vi "Zuordnungstabelle Spaltenbezeichnungen.vi"(11 "Anzahl der Stellungen (10)":i16=10) -> (3 "Spaltenbezeichnungen":string[](array[string]))   [LabVIEW 2020, in "Anlagenuebersicht.lvlib" / "VisBx Anzeige.lvlib"]
doc: "Die Zuordnungstabelle hat für jede Prozessvariable eine Zeile und enthält in\n\nSpalte 0 (Stellung x):\nden bisherigen Wert der Variablen, der zB. der Stellung eines Ventils entspricht (Boolean, U8 oder Enum),\nbei Ziffernanzeigen (U16, I16, ... DBL) immer Null.\n\nSpalte 1 (steuernd):\ndie Variablen-Nummer N einer anderen Prozessvariablen, welche die Parameter einer Ziffernanzeige festlegt (steuerndes N vom Typ Boolean, U8 oder Enum). Wenn keine Steuerung der Parameter verwendet wird, ist der Wert -1.\n\nSpalte 2 (Nachkomma):\ndie Anzahl der Nachkommastellen beim Datentyp DBL, sonst 0.\n\nSpalte 3 (Stellungstyp):\n0 ... kein Stellungstyp, zB. Ziffernanzeige\n1 ... Stellungstyp (Boolean, U8 oder Enum)\n\nSpalte 4: Programmindex für x=0\nSpalte 5: Anzahl der Programm-Schritte für x=0\n\nSpalte 6: Programmindex für x=1\nSpalte 7: Anzahl der Programm-Schritte für x=1\n....\n....\nSpalte 22: Programmindex für x=9\nSpalte 23: Anzahl der Programm-Schritte für x=9"
uses:
  VisBx Anzeige.lvlib
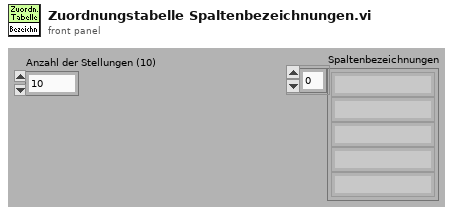
[diagram p1: front panel]
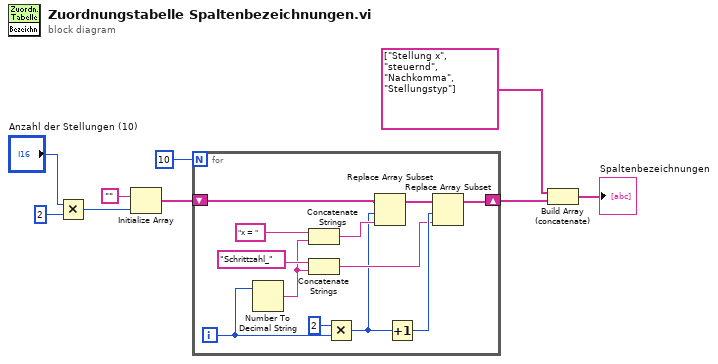
[diagram p0: block diagram]
diagram:
  n1 = Multiply(x="Anzahl der Stellungen (10)", y=i16 2) -> (x*y=w1:i16)
  n2 = Initialize Array("", w1) -> (w8:string[])
  n3 = for {
    N: 10 -> [_]
    shift-right: [w11] -> w5
    shift-left: w8 -> [w18]
    i -> [w15]
    n4 = Number To Decimal String(number=w15) -> (decimal integer string=w19:string)  [unwired: 1 out]
    n5 = Concatenate Strings("x = ", w19) -> (w13:string)
    n6 = Concatenate Strings("Schrittzahl_", w19) -> (w12:string)
    n7 = Multiply(x=2, y=w15) -> (x*y=w10:i32)
    n8 = Replace Array Subset(array=w18, new element=w13, index=w10) -> (w17:string[])
    n9 = Increment(x=w10) -> (x+1=w16:i32)
    n10 = Replace Array Subset(array=w17, new element=w12, index=w16) -> (w11:string[])
  }
  n11 = Build Array (concatenate)(string[] ["Stellung x", "steuernd", "Nachkomma", "Stellungstyp"], w5) -> (→"Spaltenbezeichnungen":string[])
